vi "Find Resource.vi"(6 "Force pass (Debugging)":bool, 8 "error in (no error)":errorcluster, 10 "Known Device IDN":string[](array[string])) -> (0 "error out":errorcluster, 1 "Return IDN":string, 2 "Resource Name":string)   [LabVIEW 2017]
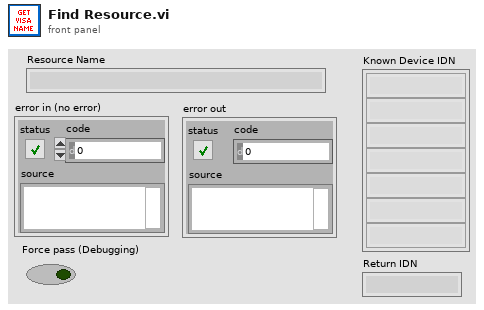
[diagram p1: front panel]
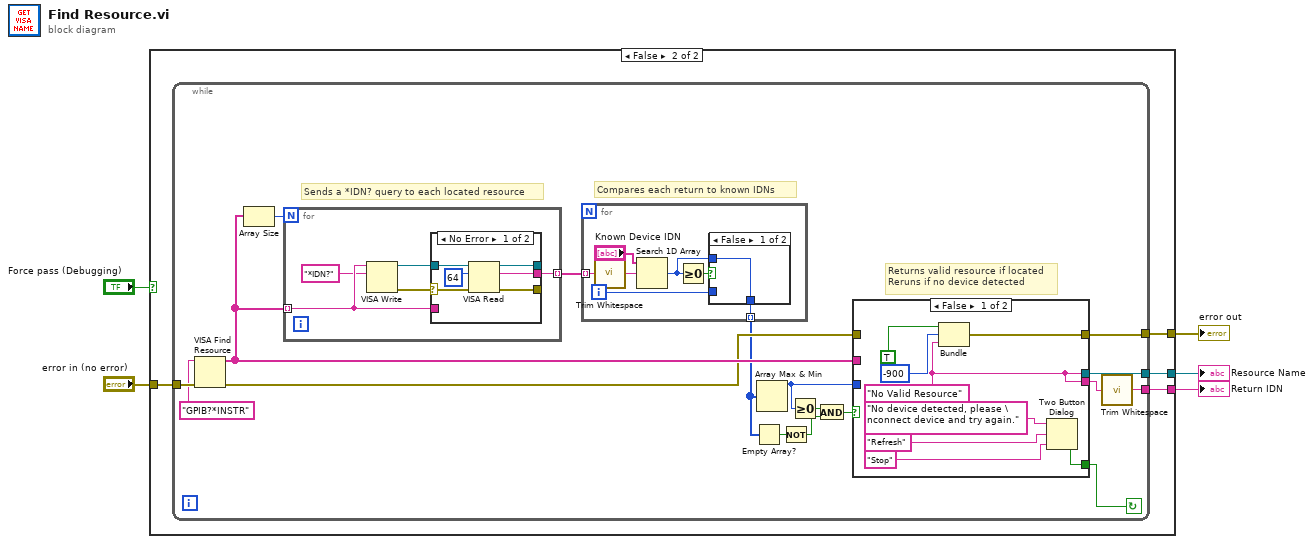
[diagram p0: block diagram]
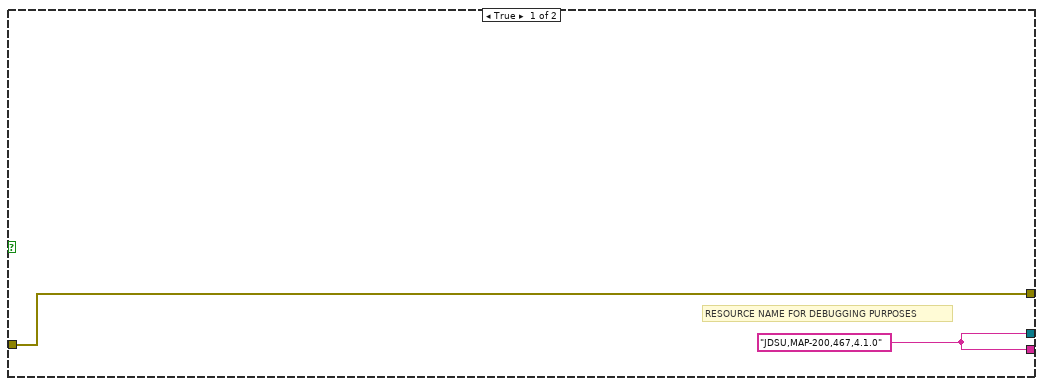
[diagram p2: hidden frame]
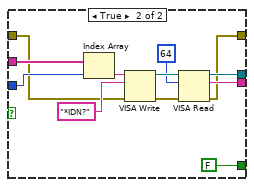
[diagram p3: hidden frame]
diagram:
  n1 = case shown="False" "Force pass (Debugging)" {
    tunnel: "error in (no error)" -> [w7 w11]
    tunnel: [w7 w10] -> w4
    tunnel: [w6 w9] -> w3
    tunnel: [w6 w8] -> w2
    frame True {
      w6 = "JDSU,MAP-200,467,4.1.0"
      # "RESOURCE NAME FOR DEBUGGING PURPOSES"
    }
    frame False {
      n2 = while {
        tunnel: [w20] -> w9
        tunnel: [w23] -> w8
        tunnel: w11 -> [w26]
        tunnel: [w21] -> w10
        stop <- w12 continue-if-true
        # "Returns valid resource if located\nReruns if no device detected"
        # "Compares each return to known IDNs"
        # "Sends a *IDN? query to each located resource"
        n3 = VISA Find Resource(8:w26, 11:"GPIB?*INSTR") -> (0:w22:errorcluster, 3:w25:string[])  [unwired: 1 in, 1 out]
        n4 = Array Size(array=w25) -> (size(s)=w28:i32)
        n5 = for {
          N: w28 -> [_]
          tunnel: w25 -> [w60] mode=indexing
          tunnel: [w58] -> w27 mode=indexing
          n6 = VISA Write(VISA resource name=w60, write buffer="*IDN?") -> (VISA resource name out=w62:refnum<visa-resource-name>, error out=w61:errorcluster)  [unwired: 1 in, 1 out]
          n7 = case shown="No Error" w61 {
            selector: w61 -> [w66 w70]
            tunnel: w62 -> [w68 w69]
            tunnel: w60 -> [_ _]
            tunnel: [w67 _] -> w58
            tunnel: [w65 w69] -> _
            tunnel: [w63 w70] -> _
            frame No Error {
              n8 = VISA Read(VISA resource name=w68, byte count=u32 64, error in (no error)=w66) -> (VISA resource name out=w65:refnum<visa-resource-name>, read buffer=w67:string, error out=w63:errorcluster)  [unwired: 1 out]
            }
            frame Error {
            }
          }
        }
        n9 = for {
          tunnel: w27 -> [w50] mode=indexing
          tunnel: [w52] -> w17 mode=indexing
          i -> [w54]
          n10 = call <vilib>:"Trim Whitespace.vi"("string"=w50) -> ("trimmed string"=w49:string)  [unwired: 1 in]
          n11 = Search 1D Array(1D array="Known Device IDN", element=w49) -> (index of element=w53:i32)  [unwired: 1 in]
          n12 = Greater Or Equal To 0?(x=w53) -> (x >= 0?=w55:bool)
          n13 = case shown="False" w55 {
            tunnel: w54 -> [_ w57]
            tunnel: [w56 w57] -> w52
            tunnel: w53 -> [w56 _]
            frame False {
            }
            frame True {
            }
          }
        }
        n14 = Empty Array?(array=w17) -> (empty?=w16:bool)
        n15 = Array Max & Min(array=w17) -> (max value=w24:i32)  [unwired: 3 out]
        n16 = Not(x=w16) -> (.not. x?=w15:bool)
        n17 = Greater Or Equal To 0?(x=w24) -> (x >= 0?=w14:bool)
        n18 = And(x=w14, y=w15) -> (x .and. y?=w13:bool)
        n19 = case shown="False" w13 {
          tunnel: w22 -> [_ w45]
          tunnel: w25 -> [_ w48]
          tunnel: w24 -> [_ w47]
          tunnel: [w34 w38] -> w21
          tunnel: [w33 w40] -> w23
          tunnel: [w33 w39] -> w19
          tunnel: [w29 FALSE] -> w12
          frame False {
            w33 = "No Valid Resource"
            n20 = Bundle(TRUE, -900, w33) -> (w34:errorcluster)  [unwired: 1 in]
            n21 = Two Button Dialog(message="No device detected, please \nconnect device and try again.", 1:"Stop", 2:"Refresh") -> (T button?=w29:bool)
          }
          frame True {
            n22 = Index Array(array=w48, index=w47) -> (element=w44:string)
            n23 = VISA Write(VISA resource name=w44, write buffer="*IDN?", error in (no error)=w45) -> (VISA resource name out=w43:refnum<visa-resource-name>, error out=w42:errorcluster)  [unwired: 1 out]
            n24 = VISA Read(VISA resource name=w43, byte count=u32 64, error in (no error)=w42) -> (VISA resource name out=w40:refnum<visa-resource-name>, read buffer=w39:string, error out=w38:errorcluster)  [unwired: 1 out]
          }
        }
        n25 = call <vilib>:"Trim Whitespace.vi"("string"=w19) -> ("trimmed string"=w20:string)  [unwired: 1 in]
      }
    }
  }
  "error out" <- w4
  "Resource Name" <- w2
  "Return IDN" <- w3
